vi "Application_SaveProject.vi"(8 "error in (no error)":errorcluster, 10 "Exclude Dependencies? (F)":bool, 11 "Project in":refnum<vi>) -> (0 "error out":errorcluster, 3 "Project out":refnum<vi>)   [LabVIEW 2016]
panel:
  out "Array":errorcluster[](array[cluster])
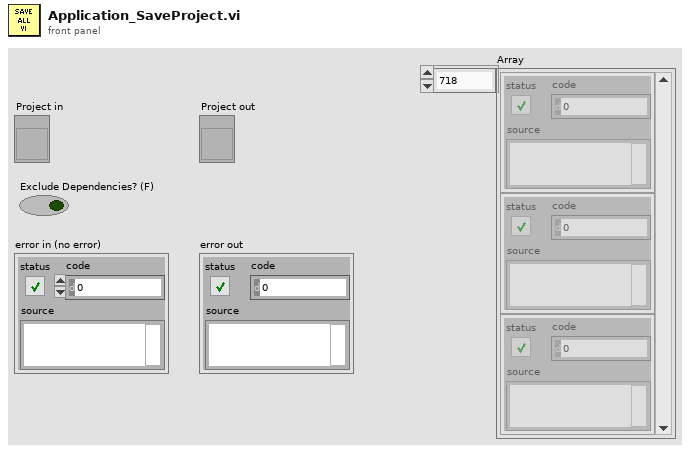
[diagram p1: front panel]
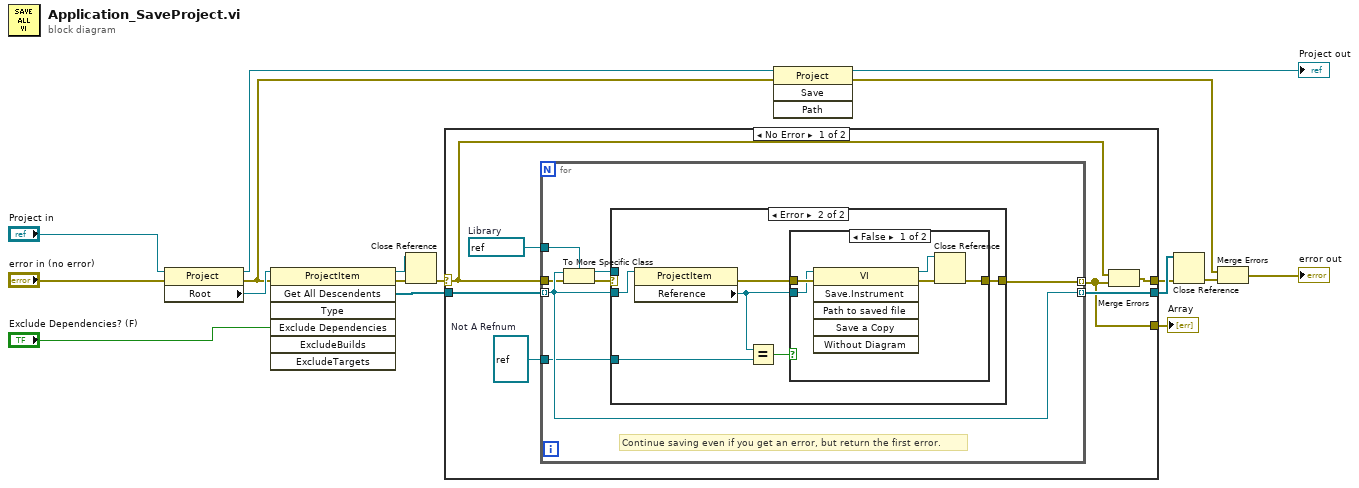
[diagram p0: block diagram]
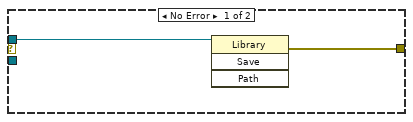
[diagram p2: hidden frame]
diagram:
  n1 = property class="Project"(reference="Project in", error in="error in (no error)") -> (reference out=w13:refnum<vi>, error out=w3:errorcluster, "Root"=w12:refnum<vi>)
  n2 = invoke class="ProjectItem" method="Get All Descendents"(reference=w12, error in=w3, "Exclude Dependencies"="Exclude Dependencies? (F)") -> (reference out=w14:refnum<vi>, error out=w15:errorcluster, "All Descendents"=w16:refnum<vi>[])  [unwired: 4 in, 4 out]
  n3 = Close Reference(reference=w14, error in (no error)=w15) -> (error out=w8:errorcluster)
  n4 = case shown="No Error" w8 {
    selector: w8 -> [w19 w47]
    tunnel: [w24 w46] -> w17
    tunnel: w16 -> [w23 w46]
    tunnel: [w20 w47] -> w7
    tunnel: [w18 _] -> w1
    frame No Error {
      w21 = refnum<vi> refnum  # Library
      w22 = refnum<vi> refnum  # Not A Refnum
      n5 = for {
        tunnel: w23 -> [w29] mode=indexing
        tunnel: [w29] -> w24 mode=indexing
        tunnel: w22 -> [w28]
        tunnel: [w27] -> w18 mode=indexing
        tunnel: w21 -> [w26]
        tunnel: w19 -> [w25]
        # "Continue saving even if you get an error, but return the first error."
        n6 = To More Specific Class(target class=w26, reference=w29, error in=w25) -> (specific class reference=w31:refnum<vi>, error out=w30:errorcluster)
        n7 = case shown="Error" w30 {
          tunnel: w31 -> [w33 _]
          tunnel: [w32 w35] -> w27
          tunnel: w29 -> [_ w38]
          tunnel: w28 -> [_ w34]
          frame No Error {
            n8 = invoke class="Library" method="Save"(reference=w33) -> (error out=w32:errorcluster)  [unwired: 3 in, 3 out]
          }
          frame Error {
            n9 = property class="ProjectItem"(reference=w38) -> (error out=w39:errorcluster, "Reference"=w36:refnum<vi>)  [unwired: 1 in, 1 out]
            n10 = Equal?(x=w36, y=w34) -> (x = y?=w37:bool)
            n11 = case shown="False" w37 {
              tunnel: w39 -> [w44 w45]
              tunnel: [w40 w45] -> w35
              tunnel: w36 -> [w43 _]
              frame False {
                n12 = invoke class="VI" method="Save.Instrument"(reference=w43, error in=w44) -> (reference out=w42:refnum<vi>, error out=w41:errorcluster)  [unwired: 4 in, 4 out]
                n13 = Close Reference(reference=w42, error in (no error)=w41) -> (error out=w40:errorcluster)
              }
              frame True {
                # "Does not return an error\nif no VI reference available."
              }
            }
          }
        }
      }
      n14 = Merge Errors(w19, w18) -> (w20:errorcluster)
    }
    frame Error {
    }
  }
  "Array" <- w1
  n15 = invoke class="Project" method="Save"(reference=w13, error in=w3) -> (reference out=→"Project out":refnum<vi>, error out=w5:errorcluster)  [unwired: 2 in, 2 out]
  n16 = Close Reference(reference=w17, error in (no error)=w7) -> (error out=w6:errorcluster)
  n17 = Merge Errors(w5, w6) -> (→"error out":errorcluster)
